vi "ExtractFloorplan.vi"(4 "FaceArray":T2(array[cluster]) {"zNorm" format="%.2f"; "yNorm" format="%.2f"; "xNorm" format="%.2f"; "zVert" format="%^#_6g"; "yVert" format="%^#_6g"; "xVert" format="%^#_6g"}) -> (1 "FloorplanArray":T2(array[cluster]) {"zNorm" format="%.2f"; "yNorm" format="%.2f"; "xNorm" format="%.2f"; "zVert" format="%^#_6g"; "yVert" format="%^#_6g"; "xVert" format="%^#_6g"})   [LabVIEW 2011]
panel:
  out "LastRow":bool=TRUE
  out "Array":string[](array[string])
  out "VertexCluster":T1 {"zNorm" format="%.2f"; "yNorm" format="%.2f"; "xNorm" format="%.2f"; "zVert" format="%^#_6g"; "yVert" format="%^#_6g"; "xVert" format="%^#_6g"}
  out "CurrentRow":i32
  out "CurrentMinZ":dbl=inf
  out "CurrentBuildIndex":u32
  out "Loop":i32
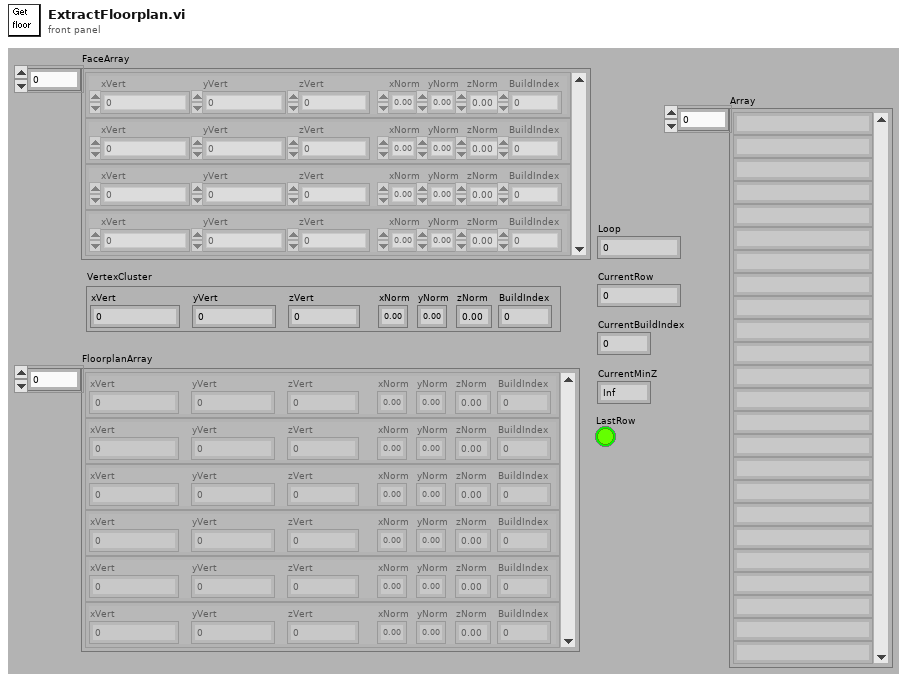
[diagram p1: front panel]
types:
  T1 = cluster{"xVert":dbl, "yVert":dbl, "zVert":dbl, "xNorm":dbl, "yNorm":dbl, "zNorm":dbl, "BuildIndex":u32}
  T2 = cluster{"xVert":dbl, "yVert":dbl, "zVert":dbl, "xNorm":dbl, "yNorm":dbl, "zNorm":dbl, "BuildIndex":u32}[]
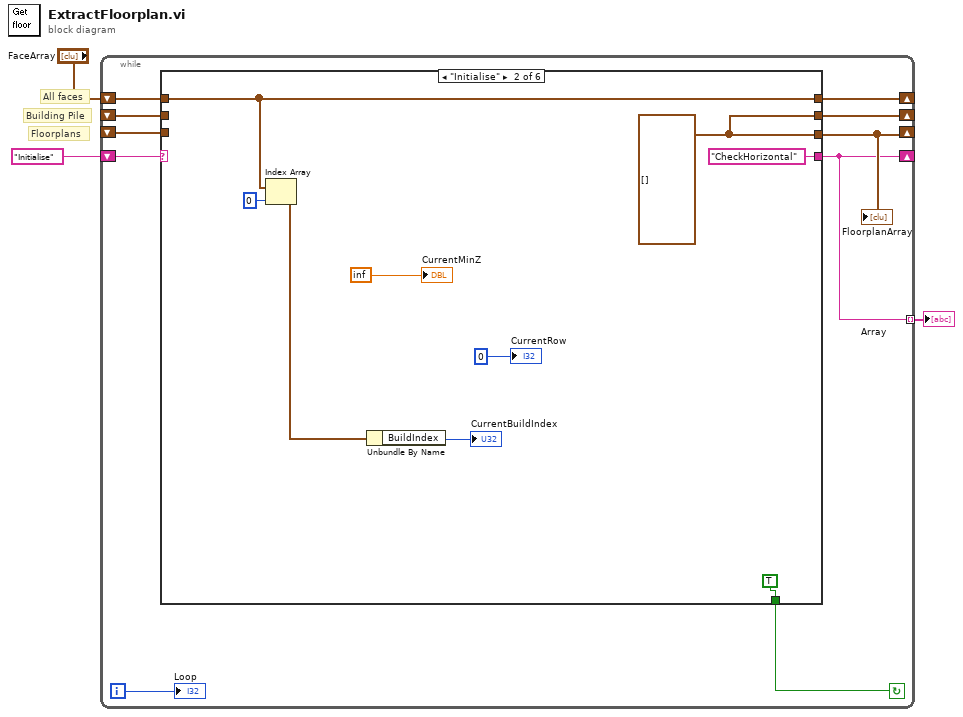
[diagram p0: block diagram]
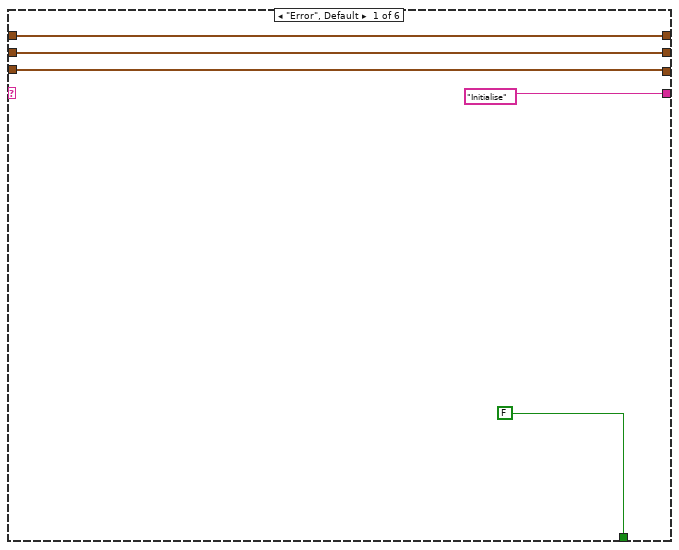
[diagram p2: hidden frame]
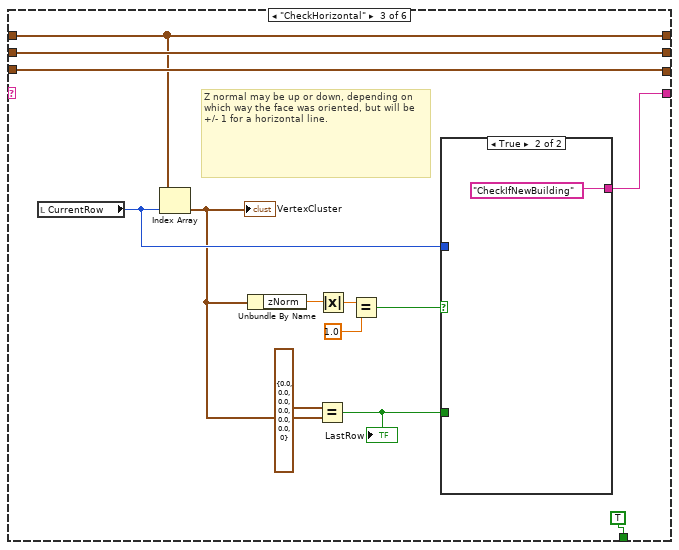
[diagram p3: hidden frame]
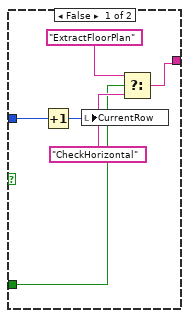
[diagram p4: hidden frame]
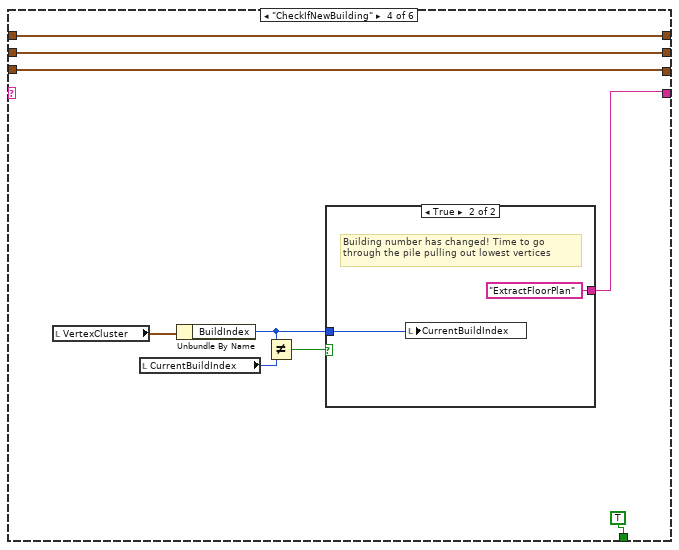
[diagram p5: hidden frame]
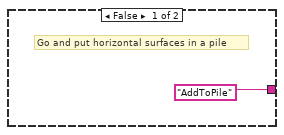
[diagram p6: hidden frame]
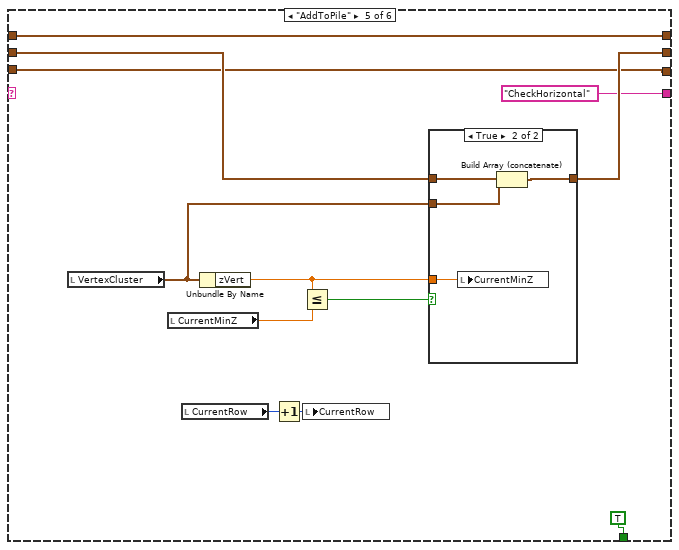
[diagram p7: hidden frame]
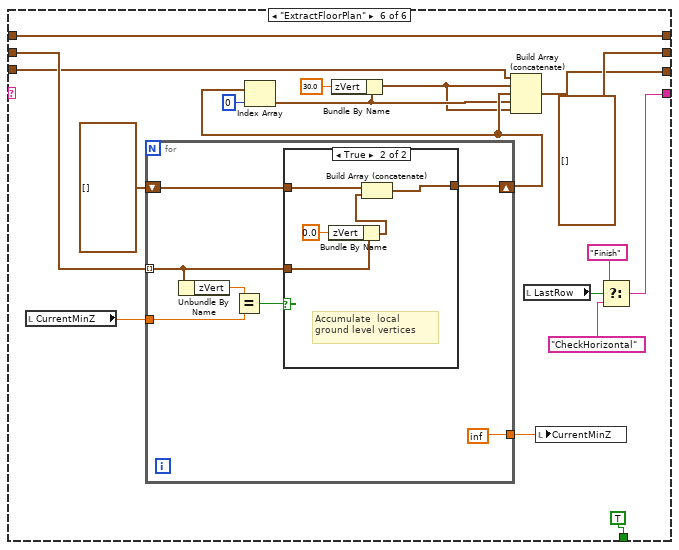
[diagram p9: hidden frame]
diagram:
  # "Floorplans"
  # "Building Pile"
  # "All faces"
  n1 = while {
    shift-right: [w6] -> _
    shift-left: "Initialise" -> [w13]
    shift-right: [w5] -> _
    shift-left: _ -> [w4]
    shift-right: [w7] -> _
    shift-left: _ -> [w11]
    shift-right: [w8] -> _
    shift-left: "FaceArray" -> [w10]
    tunnel: [w6] -> w2 mode=indexing
    i -> [w12]
    stop <- w9 continue-if-true
    n2 = case shown="\"Initialise\"" w13 {
      tunnel: ["Initialise" "CheckHorizontal" w36 w48 "CheckHorizontal" w88] -> w6
      tunnel: w10 -> [w14 w22 w38 w52 w62 w91]
      tunnel: [w17 w24 w40 w55 w70 T2 []] -> w5
      tunnel: w4 -> [w17 _ w40 w55 w69 w94]
      tunnel: w11 -> [w16 _ w39 w54 w66 w83]
      tunnel: [w16 w24 w39 w54 w66 w80] -> w7
      tunnel: [FALSE TRUE TRUE TRUE TRUE TRUE] -> w9
      tunnel: [w14 w22 w38 w52 w62 w91] -> w8
      frame "Error", Default {
      }
      frame "Initialise" {
        w24 = T2 []
        n3 = Index Array(array=w22, index=0) -> (element=w20:T1)
        n4 = Unbundle By Name(w20) -> ("BuildIndex"=→"CurrentBuildIndex":u32)
        "CurrentRow" <- 0 ("BuildingIndex")
        "CurrentMinZ" <- inf
      }
      frame "CheckHorizontal" {
        # "Z normal may be up or down, depending on which way the face was oriented, but will be  +/- 1 for a horizontal line."
        n5 = local read "CurrentRow"() -> (w37:i32)
        n6 = Index Array(array=w38, index=w37) -> (element=w29:T1)
        "VertexCluster" <- w29
        n7 = Unbundle By Name(w29) -> ("zNorm"=w34:dbl)
        n8 = Equal?(x=T1 {"xVert"=0.0, "yVert"=0.0, "zVert"=0.0, "xNorm"=0.0, "yNorm"=0.0, "zNorm"=0.0, "BuildIndex"=0} ("element"), y=w29) -> (x = y?=w28:bool)
        "LastRow" <- w28
        n9 = Absolute Value(x=w34) -> (abs(x)=w33:dbl)
        n10 = Equal?(x=w33, y=1.0) -> (x = y?=w32:bool)
        n11 = case shown="True" w32 {
          tunnel: w37 -> [w46 _]
          tunnel: [w44 "CheckIfNewBuilding" ("t")] -> w36
          tunnel: w28 -> [w41 _]
          frame False {
            n12 = Increment(x=w46) -> (x+1=w45:i32)
            n13 = local write "CurrentRow"(w45) -> ()
            n14 = Select(t="ExtractFloorPlan", s=w41, f="CheckHorizontal") -> (s? t:f=w44:string)
          }
          frame True {
          }
        }
      }
      frame "CheckIfNewBuilding" {
        n15 = local read "VertexCluster"() -> (w51:T1)
        n16 = local read "CurrentBuildIndex"() -> (w56:u32)
        n17 = Unbundle By Name(w51) -> ("BuildIndex"=w50:u32)
        n18 = Not Equal?(x=w50, y=w56) -> (x != y?=w49:bool)
        n19 = case shown="True" w49 {
          tunnel: w50 -> [_ w59]
          tunnel: ["AddToPile" "ExtractFloorPlan"] -> w48
          frame False {
            # "Go and put horizontal surfaces in a pile"
          }
          frame True {
            # "Building number has changed! Time to go through the pile pulling out lowest vertices"
            n20 = local write "CurrentBuildIndex"(w59) -> ()
          }
        }
      }
      frame "AddToPile" {
        n21 = local read "VertexCluster"() -> (w61:T1)
        n22 = local read "CurrentMinZ"() -> (w71:dbl)
        n23 = local read "CurrentRow"() -> (w65:i32)
        n24 = Unbundle By Name(w61) -> ("zVert"=w60:dbl)
        n25 = Increment(x=w65) -> (x+1=w64:i32)
        n26 = Less Or Equal?(x=w60, y=w71) -> (x <= y?=w68:bool)
        n27 = local write "CurrentRow"(w64) -> ()
        n28 = case shown="True" w68 {
          tunnel: [w72 w76] -> w70
          tunnel: w69 -> [w72 w75]
          tunnel: w61 -> [_ w74]
          tunnel: w60 -> [_ w73]
          frame False {
            # "Don't bother adding taller stuff-less to cull later"
          }
          frame True {
            n29 = local write "CurrentMinZ"(w73) -> ()
            n30 = Build Array (concatenate)(w75, w74) -> (w76:T2)
          }
        }
      }
      frame "ExtractFloorPlan" {
        n31 = local read "CurrentMinZ"() -> (w93:dbl)
        n32 = for {
          tunnel: w94 -> [w98] mode=indexing
          tunnel: w93 -> [w100]
          shift-right: [w96] -> w81
          shift-left: T2 [] -> [w97]
          tunnel: [inf] -> w85
          n33 = Unbundle By Name(w98) -> ("zVert"=w101:dbl)
          n34 = Equal?(x=w101, y=w100) -> (x = y?=w99:bool)
          n35 = case shown="True" w99 {
            tunnel: w98 -> [_ w105]
            tunnel: w97 -> [w102 w106]
            tunnel: [w102 w107] -> w96
            frame False {
            }
            frame True {
              # "Accumulate  local ground level vertices"
              n36 = Bundle By Name(cluster=w105, "zVert"=0.0) -> (w104:T1)
              n37 = Build Array (concatenate)(w106, w104) -> (w107:T2)
            }
          }
        }
        n38 = Index Array(array=w81, index=0) -> (element=w78:T1)
        n39 = Bundle By Name(cluster=w78, "zVert"=30.0) -> (w77:T1)
        n40 = Build Array (concatenate)(w83, w77, w81, w78, w77) -> (w80:T2)
        n41 = local read "LastRow"() -> (w89:bool)
        n42 = local write "CurrentMinZ"(w85) -> ()
        n43 = Select(t="Finish", s=w89, f="CheckHorizontal") -> (s? t:f=w88:string)
      }
    }
    "FloorplanArray" <- w7
    "Loop" <- w12
  }
  "Array" <- w2
